vi "catapultLoop.vi"   [LabVIEW 2017]
uses:
  <vilib>/Platform/TimedLoop/XDataNode/timing_clust.ctl
  <vilib>/Platform/TimedLoop/XDataNode/nitl_modes.ctl
  <vilib>/Platform/TimedLoop/XDataNode/wakeup.ctl
  catapultEnum.ctl
  <userlib>/836-Library/Pneumatics/Support_Code/Pneumatics_Command.ctl
  <userlib>/836-Library/Pneumatics/Support_Code/Pneumatics_Status.ctl
  <userlib>/836-Library/Pneumatics/Support_Code/Pneumatics_Command_Set_Periodic.vi
  <vilib>/platform/TimedLoop/XDataNode/XDataNode.xnode
  <vilib>/Platform/TimedLoop/XDataNode/XDNodeRunTimeDep.lvlib
types:
  T1 = typedef "XDNodeRunTimeDep.lvlib/timing_clust.ctl" = cluster{"Expected End [f-1]":u64, "Actual End [f-1]":u64, "Finished Late? [f-1]":bool, "Expected End [i-1]":u64, "Actual End [i-1]":u64, "Finished Late? [i-1]":bool, "Expected Start [i]":u64, "Actual Start [i]":u64, "Expected Start [f]":u64, "Actual Start [f]":u64, "Source Name":string, "Structure Name":string, "Period":i64, "Deadline":i64, "Offset":i64, "Start":i64, "Priority":i32, "Timeout":i32, "Mode":T2, "Wakeup Reason":T3, "Error":errorcluster, "Source Type":string, "Secondary Source Type":string, "Global End Time":u64, "Global Start Time":u64, "Frame Duration":u64, "Iteration Duration":u64, "Assigned CPU":i32, "I/O Scan Engine Mode":u32}
  T2 = typedef "XDNodeRunTimeDep.lvlib/nitl_modes.ctl" = enum32{"No Change", "Process missed periods, maintain original phase", "Discard missed periods, maintain original phase", "Process missed periods, ignore original phase", "Discard missed periods, ignore original phase"}
  T3 = typedef "XDNodeRunTimeDep.lvlib/wakeup.ctl" = enum32{"Normal", "Aborted", "Asynchronous wakeup", "Timing source error", "Timed loop error", "Timeout"}
  T4 = typedef "Pneumatics_Command.ctl" = enum16{"Nothing", "Forward", "Reverse", "Toggle"}
  T5 = typedef "catapultEnum.ctl" = enum16{"catapultBall", "doNothing"}
  T6 = cluster{"Command":refnum<notifier>, "Status":refnum<queue>}
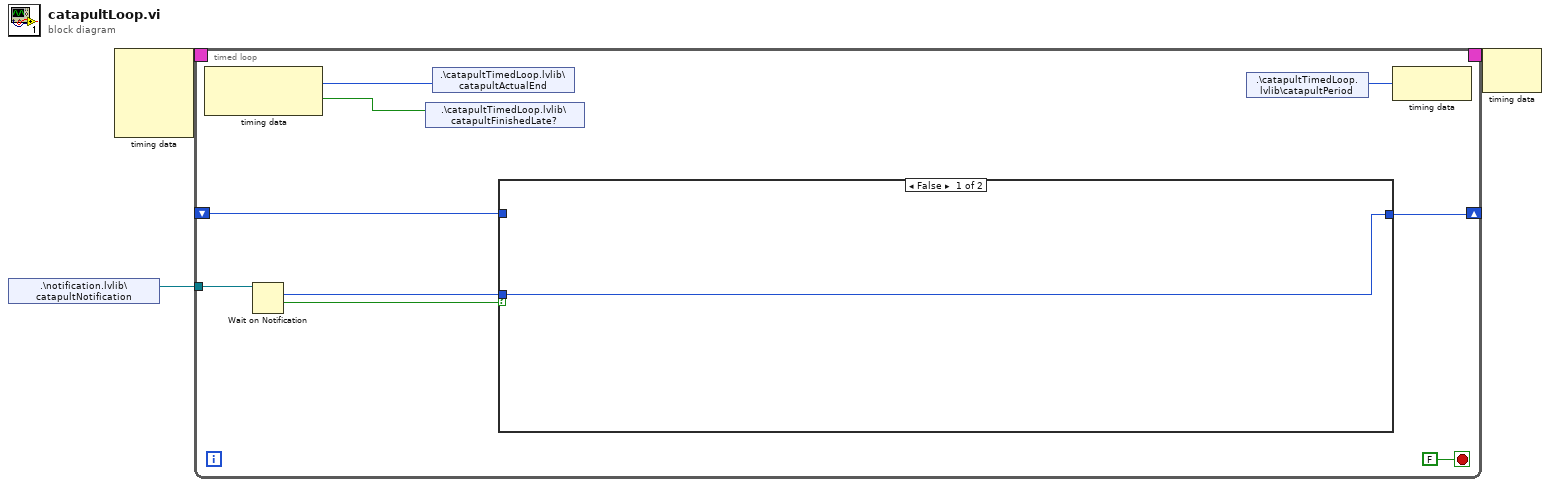
[diagram p0: block diagram]
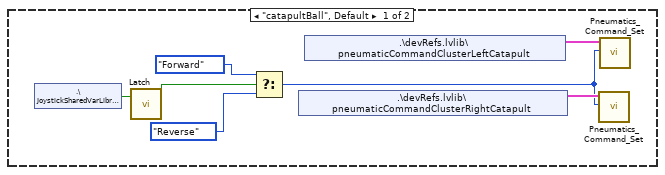
[diagram p3: hidden frame]
diagram:
  n1 = shared-variable ".\\notification.lvlib\\catapultNotification"() -> (w1:refnum<notifier>)  [unwired: 1 in, 1 out]
  n2 = node-c288() -> (w3:T1)  [unwired: 4 in]
  n3 = timed-loop {
    timing: w3 -> [_]
    timing-out: [_] -> w2
    tunnel: w1 -> [w8]
    shift-right: [w5] -> _
    shift-left: _ -> [w4]
    stop <- FALSE stop-if-true
    n4 = node-c288() -> (w11:i64, w10:bool)  [unwired: 1 in]
    n5 = Wait on Notification(notifier=w8) -> (notification=w6:T5, timed out?=w7:bool)  [unwired: 3 in, 2 out]
    n6 = shared-variable ".\\catapultTimedLoop.lvlib\\catapultFinishedLate?"(w10) -> ()  [unwired: 1 in, 1 out]
    n7 = shared-variable ".\\catapultTimedLoop.lvlib\\catapultActualEnd"(w11) -> ()  [unwired: 1 in, 1 out]
    n8 = case shown="False" w7 {
      tunnel: w6 -> [w13 _]
      tunnel: [w13 w14] -> w5
      tunnel: w4 -> [_ w14]
      frame False {
      }
      frame True {
        n9 = case shown="\"doNothing\"" w14 {
          frame "catapultBall", Default {
            n10 = shared-variable ".\\JoystickSharedVarLibrary.lvlib\\aButton"() -> (w15:bool)  [unwired: 1 in, 1 out]
            n11 = call <userlib>:"Latch.vi"("In"=w15) -> ("Out"=w17:bool)  [unwired: 1 in]
            n12 = Select(t=Pneumatics_Command."Forward" ("Solenoid Command"), s=w17, f=Pneumatics_Command."Reverse" ("Solenoid Command")) -> (s? t:f=w16:T4)
            n13 = shared-variable ".\\devRefs.lvlib\\pneumaticCommandClusterRightCatapult"() -> (w20:T6)  [unwired: 1 in, 1 out]
            n14 = shared-variable ".\\devRefs.lvlib\\pneumaticCommandClusterLeftCatapult"() -> (w21:T6)  [unwired: 1 in, 1 out]
            n15 = call-poly <userlib>:"Pneumatics_Command_Set.vi"("Solenoid Command"=w16, "Cluster"=w20) -> ()  [unwired: 9 in, 1 out]
            n16 = call-poly <userlib>:"Pneumatics_Command_Set.vi"("Solenoid Command"=w16, "Cluster"=w21) -> ()  [unwired: 9 in, 1 out]
          }
          frame "doNothing" {
          }
        }
      }
    }
    n17 = shared-variable ".\\catapultTimedLoop.lvlib\\catapultPeriod"() -> (w12:i64)  [unwired: 1 in, 1 out]
    n18 = node-c288(w12) -> ()  [unwired: 1 out]
  }
  n19 = node-c288(w2) -> ()  [unwired: 1 out]
